vi "Single Shot Pulse Sequence - 2nd Setup.vi"() -> ()   [LabVIEW 2020]
uses:
  <instrlib>/niFgen/niFgen.llb/niFgen Waveform Type.ctl
  <instrlib>/niFgen/niFgen.llb/niFgen_ctl Trigger DigEdge - Edge Values (Ring).ctl
  <instrlib>/niFgen/niFgen.llb/niFgen_ctl Trigger Source Values (Ring).ctl
  <instrlib>/niFgen/niFgen.llb/niFgen Trigger Mode.ctl
  <instrlib>/niScope/Controls/niScope acquisition type.ctl
  <instrlib>/niScope/Controls/niScope trigger slope.ctl
  <instrlib>/niScope/Controls/niScope trigger source.ctl
  <instrlib>/niFgen/niFgen.llb/niFgen Output Mode.ctl
  <instrlib>/niScope/Configure/Trigger/niScope Configure Trigger Edge.vi
  <vilib>/Utility/file.llb/Read Delimited Spreadsheet (DBL).vi
  <instrlib>/niFgen/niFgen.llb/niFgen Create Waveform (DBL).vi
  <instrlib>/niFgen/niFgen.llb/niFgen Configure Digital Edge Start Trigger.vi
  <instrlib>/niScope/Acquire/Fetch/niScope Fetch Cluster.vi
panel:
  in  "HP Amplifier":enum16{"PE15A4017", "ZHL-1-2W-S+", "ZHL-5W-1X+"}(ring)=enum."ZHL-1-2W-S+"
  in  "Larmor Frequency":dbl=27320000.0 caption="Frequency" format="%.4p"
  in  "Pulse Train File":path=path "C:/Users/localuser/OneDrive - University of South Carolina/NMR Research/MATLAB/7 us 90 Degree - 1.25 ms Tau - 3 Pulses.txt"
  out "Pulse Echo":waveform(dbl)(graph)={"t0"=timestamp(0 s since 1904-01-01), "dt"=3.3333333333333333e-06, "Y"=array[1500 elements]} caption="Waveform Graph"
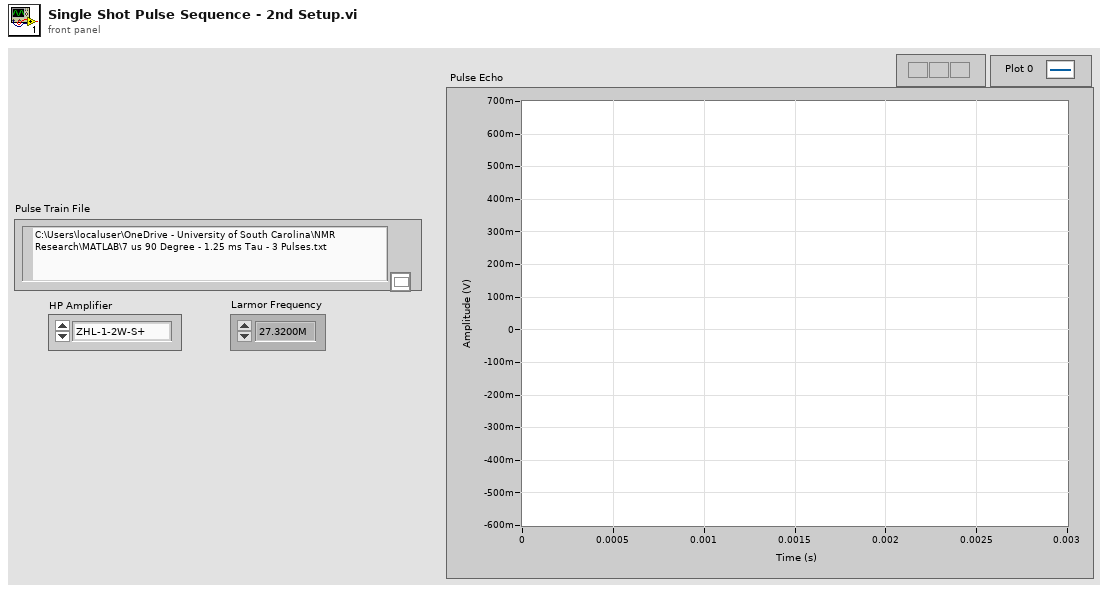
[diagram p1: front panel]
types:
  T1 = typedef "niFgen Output Mode.ctl" = u32
  T2 = typedef "niScope trigger source.ctl" = string
  T3 = typedef "niScope trigger slope.ctl" = i32
  T4 = typedef "niScope acquisition type.ctl" = i32
  T5 = typedef "niFgen Trigger Mode.ctl" = i32
  T6 = typedef "niFgen_ctl Trigger Source Values (Ring).ctl" = string
  T7 = typedef "niFgen_ctl Trigger DigEdge - Edge Values (Ring).ctl" = i32
  T8 = typedef "niFgen Waveform Type.ctl" = i32
  T9 = cluster{"relativeInitialX":dbl, "xIncrement":dbl, "wfm":dbl[]}
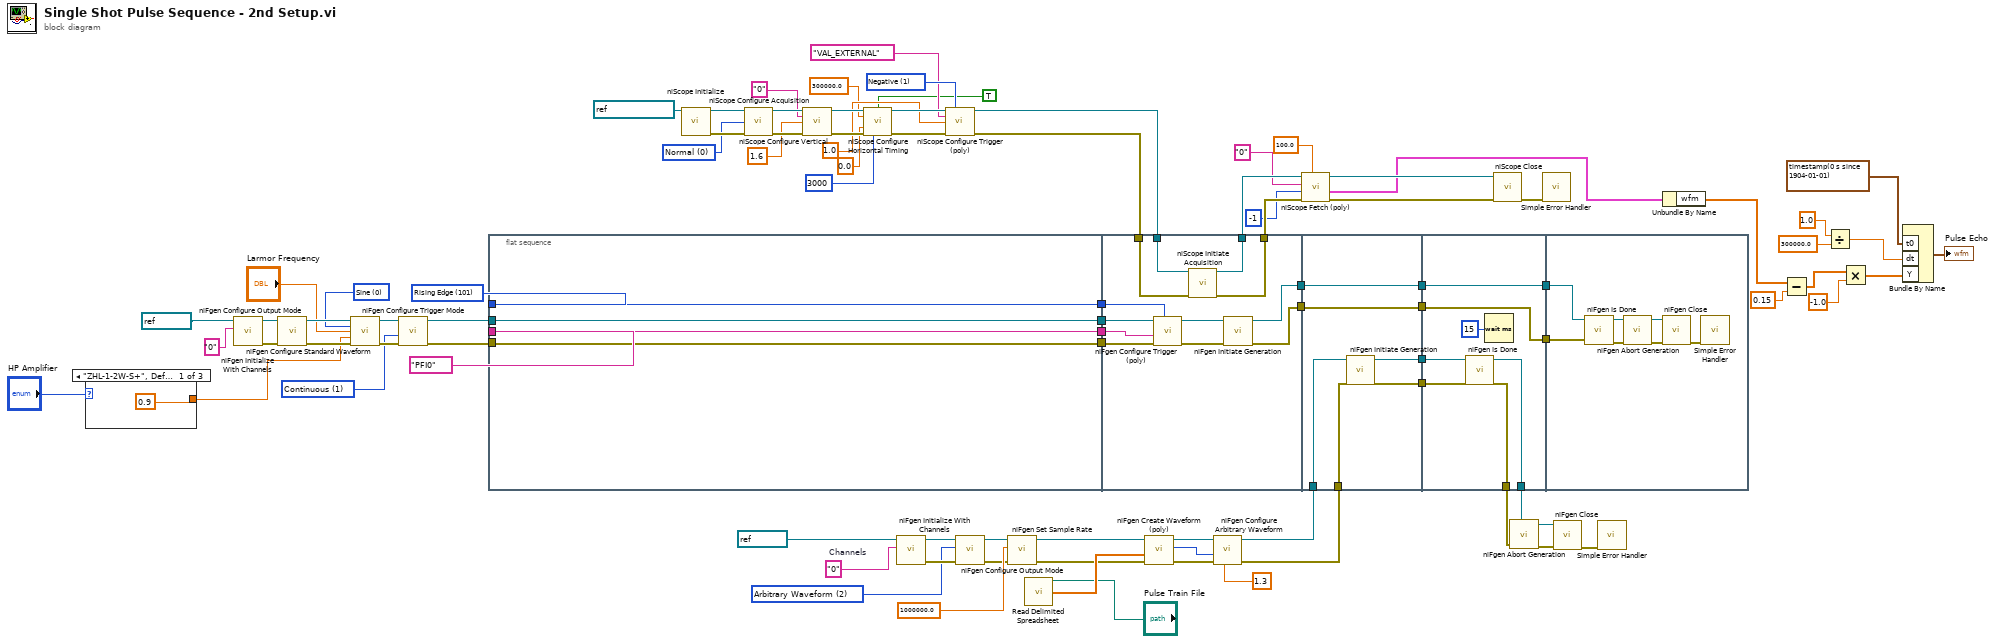
[diagram p0: block diagram]
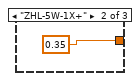
[diagram p2: hidden frame]
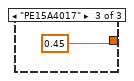
[diagram p3: hidden frame]
diagram:
  w18 = "0"  # Channels
  w17 = T1 2 items=["Standard Function", "Frequency List", "Arbitrary Waveform", "Arbitrary Sequence", "Script"] ("output mode")
  w58 = T3 1 items=["Positive", "Negative"] ("trigger slope")
  w59 = T4 0 items=["Normal"=0, "Flex Res"=1, "DDC"=3] ("acquisition Type")
  w71 = T5 1 items=["Single", "Continuous", "Stepped", "Burst"] ("Trigger Mode (default: 1=continuous)")
  w75 = T7 101 items=["Rising Edge"=101, "Falling Edge"=102] ("Edge (Rising)")
  w76 = T8 0 items=["Sine", "Square", "Triangle", "Ramp Up", "Ramp Down", "DC", "Noise", "User"] ("Waveform")
  n1 = case shown="\"ZHL-1-2W-S+\", Default" "HP Amplifier" {
    tunnel: [0.9 ("Amplitude") 0.35 ("Amplitude") 0.45 ("Amplitude")] -> w5
    frame "ZHL-1-2W-S+", Default {
    }
    frame "ZHL-5W-1X+" {
    }
    frame "PE15A4017" {
    }
  }
  n2 = call <instrlib>:"niFgen Initialize With Channels.vi"("Channel Name"="0", "Resource Name"=refnum<k15> "Dev1" ("Sine Wave Module")) -> ("error out"=w81:errorcluster, "Instrument Handle Out"=w84:refnum<k15>)  [unwired: 8 in]
  n3 = call <instrlib>:"niFgen Configure Output Mode.vi"("error in (no error)"=w81, "Instrument Handle"=w84) -> ("error out"=w80:errorcluster, "Instrument Handle Out"=w83:refnum<k15>)  [unwired: 7 in]
  n4 = call <instrlib>:"niFgen Configure Standard Waveform.vi"("Instrument Handle"=w83, "Waveform"=w76, "Frequency"="Larmor Frequency", "Amplitude"=w5, "error in (no error)"=w80) -> ("Instrument Handle Out"=w82:refnum<k15>, "error out"=w79:errorcluster)  [unwired: 9 in]
  n5 = call <instrlib>:"niFgen Configure Trigger Mode.vi"("error in (no error)"=w79, "Trigger Mode (default: 1=continuous)"=w71, "Instrument Handle"=w82) -> ("error out"=w74:errorcluster, "Instrument Handle Out"=w72:refnum<k15>)  [unwired: 7 in]
  n6 = flat-sequence {
    tunnel: w72 -> [w96]
    tunnel: T6 "PFI0" ("Source") -> [w97]
    tunnel: w74 -> [w98]
    tunnel: w75 -> [w99]
    tunnel: [w99] -> w4
    tunnel: [w98] -> w3
    tunnel: [w97] -> w2
    tunnel: [w96] -> w1
    tunnel: w52 -> [w105]
    tunnel: w51 -> [w104]
    tunnel: [w103] -> w50
    tunnel: [w102] -> w49
    tunnel: [w101] -> w92
    tunnel: [w100] -> w91
    tunnel: w4 -> [w110]
    tunnel: w3 -> [w109]
    tunnel: w2 -> [w108]
    tunnel: w1 -> [w107]
    tunnel: w16 -> [w117]
    tunnel: w15 -> [w116]
    tunnel: [w115] -> w90
    tunnel: [w114] -> w89
    tunnel: [w113] -> w88
    tunnel: w92 -> [w113]
    tunnel: [w112] -> w87
    tunnel: w91 -> [w112]
    tunnel: [w123] -> w70
    tunnel: [w122] -> w69
    tunnel: w90 -> [w121]
    tunnel: w89 -> [w120]
    tunnel: [w119] -> w86
    tunnel: w88 -> [w119]
    tunnel: [w118] -> w85
    tunnel: w87 -> [w118]
    tunnel: w86 -> [w126]
    tunnel: w85 -> [w125]
    frame #0 {
    }
    frame #1 {
      n7 = call-poly <instrlib>:"niFgen Configure Trigger (poly).vi"("Edge (Rising)"=w110, "error in (no error)"=w109, "Source"=w108, "Instrument Handle"=w107) -> ("error out"=w106:errorcluster, "Instrument Handle Out"=w111:refnum<k15>)  [unwired: 6 in]
      n8 = call <instrlib>:"niScope Initiate Acquisition.vi"("instrument handle"=w105, "error in"=w104) -> ("instrument handle out"=w103:refnum<k15>, "error out"=w102:errorcluster)  [unwired: 12 in]
      n9 = call <instrlib>:"niFgen Initiate Generation.vi"("error in (no error)"=w106, "Instrument Handle"=w111) -> ("error out"=w100:errorcluster, "Instrument Handle Out"=w101:refnum<k15>)  [unwired: 8 in]
    }
    frame #2 {
      n10 = call <instrlib>:"niFgen Initiate Generation.vi"("error in (no error)"=w117, "Instrument Handle"=w116) -> ("error out"=w114:errorcluster, "Instrument Handle Out"=w115:refnum<k15>)  [unwired: 8 in]
    }
    frame #3 {
      n11 = call <instrlib>:"niFgen Is Done.vi"("error in (no error)"=w120, "Instrument Handle"=w121) -> ("error out"=w123:errorcluster, "Instrument Handle Out"=w122:refnum<k15>)  [unwired: 7 in, 1 out]
      n12 = Wait (ms)(milliseconds to wait=u32 15) -> ()  [unwired: 1 out]
    }
    frame #4 {
      n13 = call <instrlib>:"niFgen Is Done.vi"("error in (no error)"=w125, "Instrument Handle"=w126) -> ("error out"=w129:errorcluster, "Instrument Handle Out"=w128:refnum<k15>)  [unwired: 7 in, 1 out]
      n14 = call <instrlib>:"niFgen Abort Generation.vi"("error in (no error)"=w129, "Instrument Handle"=w128) -> ("error out"=w130:errorcluster, "Instrument Handle Out"=w131:refnum<k15>)  [unwired: 8 in]
      n15 = call <instrlib>:"niFgen Close.vi"("error in (no error)"=w130, "Instrument Handle"=w131) -> ("error out"=w127:errorcluster)  [unwired: 9 in]
      n16 = call <vilib>:"Simple Error Handler.vi"("error in (no error)"=w127) -> ()  [unwired: 4 in, 5 out]
    }
  }
  n17 = call <instrlib>:"niScope Initialize.vi"("resource name"=refnum<k15> "PXI1Slot6_2") -> ("instrument handle"=w60:refnum<k15>, "error out"=w61:errorcluster)  [unwired: 13 in]
  n18 = call <instrlib>:"niScope Configure Acquisition.vi"("instrument handle"=w60, "acquisition Type"=w59, "error in"=w61) -> ("instrument handle out"=w62:refnum<k15>, "error out"=w63:errorcluster)  [unwired: 11 in]
  n19 = call <instrlib>:"niScope Configure Vertical.vi"("instrument handle"=w62, "channels"="0", "vertical range"=1.6, "error in"=w63) -> ("instrument handle out"=w64:refnum<k15>, "error out"=w65:errorcluster)  [unwired: 10 in]
  n20 = call <instrlib>:"niScope Configure Horizontal Timing.vi"("instrument handle"=w64, "enforce realtime"=TRUE, "min sample rate"=300000.0, "reference position"=0.0, "error in"=w65, "min record length"=3000) -> ("instrument handle out"=w66:refnum<k15>, "error out"=w67:errorcluster)  [unwired: 8 in]
  n21 = call <instrlib>:"niFgen Initialize With Channels.vi"("Channel Name"=w18, "Resource Name"=refnum<k15> "Dev3" ("FGEN Resource Name 2")) -> ("error out"=w21:errorcluster, "Instrument Handle Out"=w22:refnum<k15>)  [unwired: 8 in]
  n22 = call-poly <instrlib>:"niScope Configure Trigger (poly).vi"("instrument handle"=w66, "trigger slope"=w58, "trigger source"=T2 "VAL_EXTERNAL", "trigger level"=1.0, "error in"=w67) -> ("instrument handle out"=w52:refnum<k15>, "error out"=w51:errorcluster)  [unwired: 9 in]
  n23 = call <instrlib>:"niFgen Configure Output Mode.vi"("error in (no error)"=w21, "Output Mode (default: 0=Standard Function)"=w17, "Instrument Handle"=w22) -> ("error out"=w25:errorcluster, "Instrument Handle Out"=w24:refnum<k15>)  [unwired: 6 in]
  n24 = call <instrlib>:"niFgen Set Sample Rate.vi"("error in (no error)"=w25, "Sample Rate (Samp/s)"=1000000.0 ("Sample Rate"), "Instrument Handle"=w24) -> ("error out"=w28:errorcluster, "Instrument Handle Out"=w27:refnum<k15>)  [unwired: 7 in]
  n25 = call-poly <vilib>:"Read Delimited Spreadsheet.vi"("file path (dialog if empty)"="Pulse Train File") -> ("first row"=w29:dbl[])  [unwired: 9 in, 5 out]
  n26 = call-poly <instrlib>:"niFgen Create Waveform (poly).vi"("error in (no error)"=w28, "Waveform Data Array"=w29, "Instrument Handle"=w27) -> ("error out"=w31:errorcluster, "Waveform Handle"=w32:i32, "Instrument Handle Out"=w30:refnum<k15>)  [unwired: 6 in]
  n27 = call <instrlib>:"niFgen Configure Arbitrary Waveform.vi"("Gain"=1.3, "error in (no error)"=w31, "Waveform Handle"=w32, "Instrument Handle"=w30) -> ("error out"=w16:errorcluster, "Instrument Handle Out"=w15:refnum<k15>)  [unwired: 6 in]
  n28 = call-poly <instrlib>:"niScope Fetch (poly).vi"("timeout"=100.0, "error in"=w49, "numSamples"=-1, "channels"="0", "instrument handle"=w50) -> ("error out"=w42:errorcluster, "waveform"=w40:T9, "instrument handle out"=w43:refnum<k15>)  [unwired: 3 in, 1 out]
  n29 = call <instrlib>:"niScope Close.vi"("instrument handle"=w43, "error in"=w42) -> ("error out"=w68:errorcluster)  [unwired: 13 in]
  n30 = call <instrlib>:"niFgen Abort Generation.vi"("error in (no error)"=w70, "Instrument Handle"=w69) -> ("error out"=w10:errorcluster, "Instrument Handle Out"=w11:refnum<k15>)  [unwired: 8 in]
  n31 = call <vilib>:"Simple Error Handler.vi"("error in (no error)"=w68) -> ()  [unwired: 4 in, 5 out]
  n32 = call <instrlib>:"niFgen Close.vi"("error in (no error)"=w10, "Instrument Handle"=w11) -> ("error out"=w12:errorcluster)  [unwired: 9 in]
  n33 = call <vilib>:"Simple Error Handler.vi"("error in (no error)"=w12) -> ()  [unwired: 4 in, 5 out]
  n34 = Unbundle By Name(w40) -> ("wfm"=w34:dbl[])
  n35 = Subtract(x=w34, y=0.15) -> (x-y=w9:dbl[])
  n36 = Divide(x=1.0, y=300000.0) -> (x/y=w39:dbl)
  n37 = Multiply(x=w9, y=-1.0) -> (x*y=w8:dbl[])
  n38 = Bundle By Name("t0"=timestamp(0 s since 1904-01-01), "dt"=w39, "Y"=w8) -> (→"Pulse Echo":waveform(dbl))  [unwired: 1 in]
